vi "Read U8 FIFO.vi"(8 "error in (no error)":errorcluster, 9 "Timeout (ms)":i32=100, 10 "Return Data":bool=TRUE, 11 "CIFFIFO in":refnum<class "CIF_NIChn_Fifo_U8.lvclass">) -> (0 "error out":errorcluster, 1 "timed out?":bool, 2 "U8 Data":u8[](array[numeric]), 3 "CIFFIFO out":refnum<class "CIF_NIChn_Fifo_U8.lvclass">, 4 "Header":T1)   [LabVIEW 2021, in "CIF_NIChn_Fifo_U8.lvclass"]
uses:
  CIF_NIChn_Fifo_U8.lvclass
  D:/dev/Packages/Channel_Manager/src/CIFChannels/CIFChannels.lvclass
  D:/dev/Packages/Channel_Manager/src/CIF_NIChn/NIChn/CIF_NIChn.lvclass
  ChannelCommon/typedef/FIFO Header.ctl
  CIFChannels/Typedef/Direction.ctl
  CIFChannels/Typedef/Channel State.ctl
  CIFChannels/CIFChannels.lvclass/CIFChannels.ctl
  NIChn/CIF_NIChn.lvclass/CIF_NIChn.ctl
  CIF_NIChn_Fifo_U8.lvclass/CIF_NIChn_Fifo_U8.ctl
  <vilib>/CIF Foundation/CIF Utilities/Statistics/I64/Stats_I64_CIF_U.lvclass/Stats_I64_CIF_U.ctl
  e6dc5e5d-6043-485e-a6bf-7c23d051166d.vi
  66a3f3ff-bc1e-4ae7-83d8-3035fbf2cfec.vi
  CIFChannels/Accessors/Read Channel State.vi
  CIFChannels/Accessors/Read Direction.vi
  <vilib>/CIF Foundation/CIF Utilities/Time/System Time/Get System Time.vi
  <vilib>/CIF Foundation/CIF Utilities/DataTypes/Unflatten U64.vi
  <vilib>/CIF Foundation/CIF Utilities/DataTypes/Unflatten I64.vi
  ChannelCommon/Utilities/Add Error.vi
  CIFChannels/Accessors/Write Channel State.vi
  CIFChannels/Accessors/Read Tag Disconnect Behavior.vi
  <vilib>/CIF Foundation/CIF Utilities/Statistics/I64/X1 minus X0.vi
  <vilib>/CIF Foundation/CIF Utilities/Time/System Time/LabVIEW Time to TAI Time.vi
  <vilib>/CIF Foundation/CIF Utilities/Errors/Append Error Location.vi
  <vilib>/CIF Foundation/CIF Utilities/Statistics/I64/X1 minus X0.vi/dfabcf33-0dbc-4041-80a5-3dc0c86d2989.vi
  <vilib>/CIF Foundation/CIF Utilities/Statistics/I64/X1 minus X0.vi/dfabcf33-0dbc-4041-80a5-3dc0c86d2989.vi/9eb60a9a-770f-4d2d-8b3f-8465c267ecc9.vi
  NIChn/CIF_NIChn.lvclass
  CIFChannels/CIFChannels.lvclass
  <vilib>/CIF Foundation/CIF Channels/CIFChannels/CIFChannelCore.lvlib
  ChannelCommon/ChannelCommon.lvlib
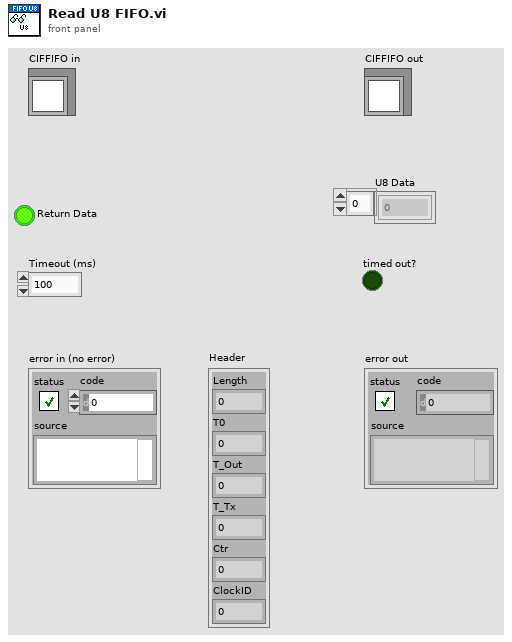
[diagram p1: front panel]
types:
  T1 = typedef "ChannelCommon.lvlib/FIFO Header.ctl" = cluster{"Length":u64, "T0":i64, "T_Out":i64, "T_Tx":i64, "Ctr":u64, "ClockID":u8}
  T2 = typedef "CIFChannels.lvclass/Channel State.ctl" = enum16{"Creating", "Disconnected", "Connecting", "Connected", "Destroyed"}
  T3 = typedef "CIFChannels.lvclass/Direction.ctl" = enum16{"Publisher", "Subscriber"}
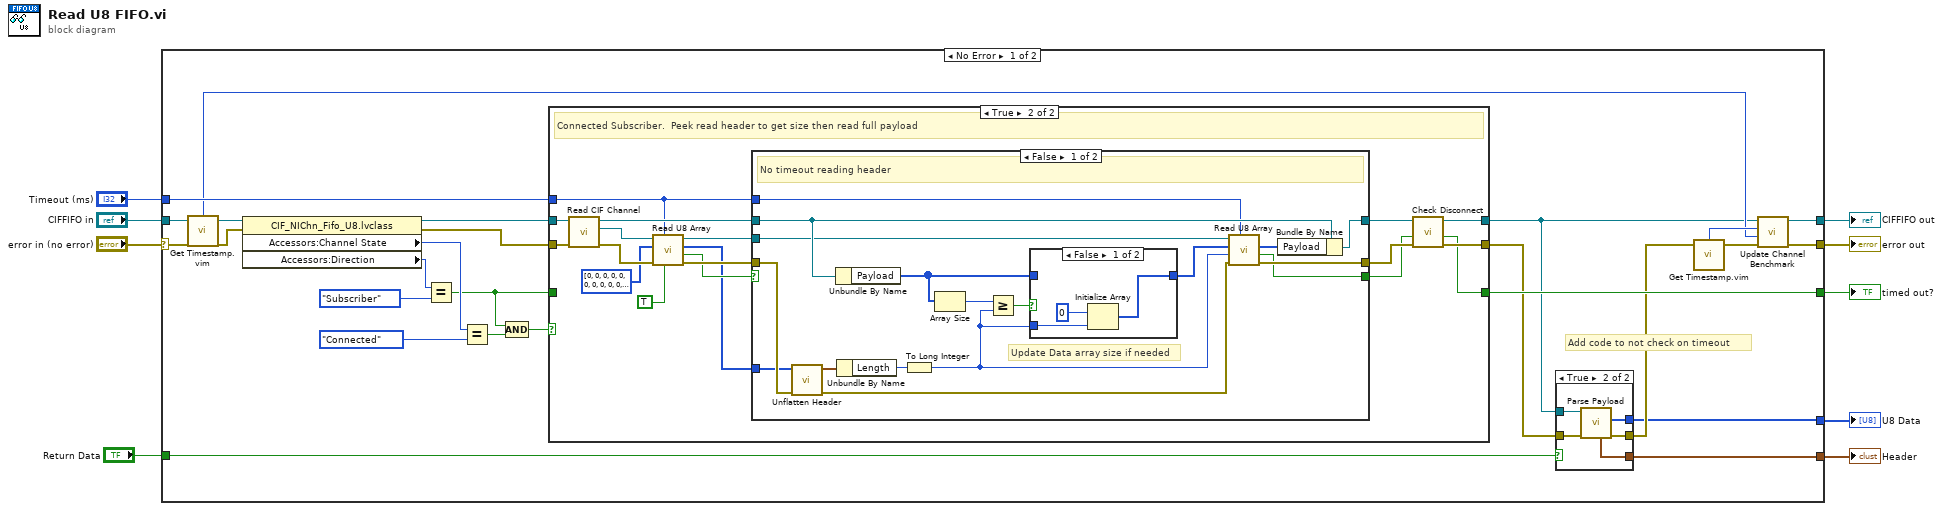
[diagram p0: block diagram]
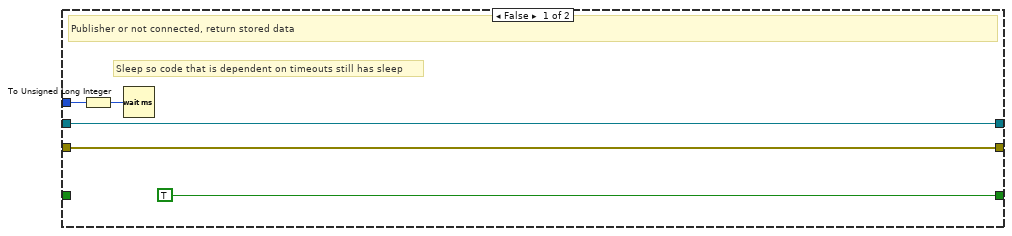
[diagram p3: hidden frame]
diagram:
  n1 = case shown="No Error" "error in (no error)" {
    selector: "error in (no error)" -> [w21 w89]
    tunnel: [w22 w89] -> w8
    tunnel: [w23 w88] -> w6
    tunnel: "CIFFIFO in" -> [w20 w88]
    tunnel: [w34 _] -> w5
    tunnel: "Timeout (ms)" -> [w24 _]
    tunnel: [w12 _] -> w3
    tunnel: [w10 _] -> w2
    tunnel: "Return Data" -> [w13 _]
    frame No Error {
      # "Add code to not check on timeout"
      n2 = call "Get Timestamp.vim"("Anything in"=w20) -> ("Time (ns)"=w17:i64, "Anything out"=w19:refnum<class "CIF_NIChn_Fifo_U8.lvclass">)  [unwired: 2 in]
      n3 = property class="CIF_NIChn_Fifo_U8.lvclass"(reference=w19, error in=w21) -> (reference out=w33:refnum<class "CIF_NIChn_Fifo_U8.lvclass">, error out=w32:errorcluster, "Accessors:Channel State"=w29:T2, "Accessors:Direction"=w31:T3)
      n4 = Equal?(x=w31, y=Direction."Subscriber") -> (x = y?=w25:bool)
      n5 = Equal?(x=w29, y=Channel_State."Connected") -> (x = y?=w27:bool)
      n6 = Compound Arithmetic op=AND(w25, w27) -> (w26:bool)
      n7 = case shown="True" w26 {
        tunnel: [TRUE ("timeout out") w56] -> w34
        tunnel: w32 -> [w44 w62]
        tunnel: w33 -> [w45 w63]
        tunnel: w25 -> [_ _]
        tunnel: [w45 w61] -> w11
        tunnel: [w44 w60] -> w16
        tunnel: w24 -> [w42 w47]
        frame False {
          # "Sleep so code that is dependent on timeouts still has sleep"
          # "Publisher or not connected, return stored data"
          n8 = To Unsigned Long Integer(number=w42) -> (unsigned 32bit integer=w41:u32)
          n9 = Wait (ms)(milliseconds to wait=w41) -> ()  [unwired: 1 out]
        }
        frame True {
          # "Connected Subscriber.  Peek read header to get size then read full payload"
          n10 = call "Read CIF Channel.vi"("error in (no error)"=w62, "CIFTag in"=w63) -> ("error out"=w57:errorcluster, "CIF Channel"=w58:refnum<k21>, "CIFTag out"=w59:refnum<class "CIF_NIChn_Fifo_U8.lvclass">)  [unwired: 7 in]
          n11 = call <vilib>:"Read U8 Array.vi"("Peek?"=TRUE, "Timeout (ms)"=w47, "error in"=w57, "U8 Array in"=u8[] [0, 0, 0, 0, 0, 0, 0, 0, 0, 0, 0, 0, 0, 0, 0, 0, 0, 0, 0, 0, 0, 0, 0, 0, 0, 0, 0, 0, 0, 0, 0, 0, 0, 0, 0, 0, 0, 0, 0, 0, 0, 0, 0, 0, 0, 0, 0, 0], "CIF Channel in"=w58) -> ("error out"=w54:errorcluster, "Timed out?"=w49:bool, "U8 Array out"=w46:u8[], "CIF Channel out"=w55:refnum<k21>)  [unwired: 3 in]
          n12 = case shown="False" w49 {
            selector: w49 -> [_ w87]
            tunnel: w59 -> [w80 w86]
            tunnel: w55 -> [w79 _]
            tunnel: w54 -> [w72 w85]
            tunnel: w46 -> [w70 _]
            tunnel: [w77 w85] -> w51
            tunnel: [w76 w86] -> w50
            tunnel: [w74 w87] -> w48
            tunnel: w47 -> [w73 _]
            frame False {
              # "Update Data array size if needed"
              # "No timeout reading header"
              n13 = call "Unflatten Header.vi"("error in (no error)"=w72, "Flattened Data in"=w70) -> ("error out"=w71:errorcluster, "Header out"=w78:T1)  [unwired: 7 in, 1 out]
              n14 = Unbundle By Name(w80) -> ("Payload"=w65:u8[])
              n15 = Unbundle By Name(w78) -> ("Length"=w75:u64)
              n16 = To Long Integer(number=w75) -> (32bit integer=w66:i32)
              n17 = Array Size(array=w65) -> (size(s)=w67:i32)
              n18 = Greater Or Equal?(x=w67, y=w66) -> (x >= y?=w68:bool)
              n19 = case shown="False" w68 {
                tunnel: w65 -> [_ w84]
                tunnel: [w83 w84] -> w64
                tunnel: w66 -> [w81 _]
                frame False {
                  n20 = Initialize Array(u8 0, w81) -> (w83:u8[])
                }
                frame True {
                }
              }
              n21 = call <vilib>:"Read U8 Array.vi"("Timeout (ms)"=w73, "error in"=w71, "Number of Elements"=w66, "U8 Array in"=w64, "CIF Channel in"=w79) -> ("error out"=w77:errorcluster, "Timed out?"=w74:bool, "U8 Array out"=w69:u8[])  [unwired: 3 in, 1 out]
              n22 = Bundle By Name(cluster=w80, "Payload"=w69) -> (w76:refnum<class "CIF_NIChn_Fifo_U8.lvclass">)
            }
            frame True {
              # "Timeout reading header"
            }
          }
          n23 = call "Check Disconnect.vi"("error in (no error)"=w51, "timeout in"=w48, "CIFTag in"=w50) -> ("error out"=w60:errorcluster, "timeout out"=w56:bool, "CIFTag out"=w61:refnum<class "CIF_NIChn_Fifo_U8.lvclass">)  [unwired: 5 in, 1 out]
        }
      }
      n24 = case shown="True" w13 {
        tunnel: w11 -> [_ w36]
        tunnel: w16 -> [w35 w40]
        tunnel: [w35 w39] -> w15
        tunnel: [_ w38] -> w10
        tunnel: [_ w37] -> w12
        frame False {
        }
        frame True {
          n25 = call "Parse Payload.vi"("error in (no error)"=w40, "CIFFIFO in"=w36) -> ("error out"=w39:errorcluster, "Data"=w38:u8[], "Header out"=w37:T1)  [unwired: 7 in]
        }
      }
      n26 = call "Get Timestamp.vim"("Anything in"=w15) -> ("Time (ns)"=w18:i64, "Anything out"=w14:errorcluster)  [unwired: 2 in]
      n27 = call "Update Channel Benchmark.vi"("error in (no error)"=w14, "X0"=w17, "X1"=w18, "CIFChannels in"=w11) -> ("error out"=w22:errorcluster, "CIFChannels out"=w23:refnum<class "CIF_NIChn_Fifo_U8.lvclass">)  [unwired: 6 in]
    }
    frame Error {
    }
  }
  "error out" <- w8
  "CIFFIFO out" <- w6
  "timed out?" <- w5
  "Header" <- w3
  "U8 Data" <- w2
